vi "GeoData.vi"() -> ()   [LabVIEW 2017] (continued)
H1\n44202\t39133\tAurora\tOH\tPortage County\tH1\n44491\t39133\tWest farmington\tOH\tPortage County\tH1\n44201\t39133\tAtwater\tOH\tPortage County\tH1\n44601\t39133\tAlliance\tOH\tPortage County\tH1\n44412\t39133\tDiamond\tOH\tPortage County\tH1\n44265\t39133\tRandolph\tOH\tPortage County\tH1\n44255\t39133\tMantua\tOH\tPortage County\tH1\n44231\t39133\tGarrettsville\tOH\tPortage County\tH1\n44288\t39133\tWindham\tOH\tPortage County\tH1\n44312\t39133\tAkron\tOH\tPortage County\tH1\n44429\t39133\tLake milton\tOH\tPortage County\tH1\n44632\t39133\tHartville\tOH\tPortage County\tH1\n44234\t39133\tHiram\tOH\tPortage County\tH1\n44224\t39133\tStow\tOH\tPortage County\tH1\n44444\t39133\tNewton falls\tOH\tPortage County\tH1\n44470\t39133\tSouthington\tOH\tPortage County\tH1\n44411\t39133\tDeerfield\tOH\tPortage County\tH1\n45003\t39135\tCollege corner\tOH\tPreble County\tH1\n45304\t39135\tArcanum\tOH\tPreble County\tH1\n45382\t39135\tWest manchester\tOH\tPreble County\tH1\n45311\t39135\tCamden\tOH\tPreble County\tH1\n45338\t39135\tLewisburg\tOH\tPreble County\tH1\n45309\t39135\tBrookville\tOH\tPreble County\tH1\n45327\t39135\tGermantown\tOH\tPreble County\tH1\n45381\t39135\tWest alexandria\tOH\tPreble County\tH1\n45064\t39135\tSomerville\tOH\tPreble County\tH1\n45320\t39135\tEaton\tOH\tPreble County\tH1\n45347\t39135\tNew paris\tOH\tPreble County\tH1\n45378\t39135\tVerona\tOH\tPreble County\tH1\n45070\t39135\tWest elkton\tOH\tPreble County\tH1\n45042\t39135\tMiddletown\tOH\tPreble County\tH1\n45056\t39135\tOxford\tOH\tPreble County\tH1\n45325\t39135\tFarmersville\tOH\tPreble County\tH1\n45321\t39135\tEldorado\tOH\tPreble County\tH1\n45330\t39135\tGratis\tOH\tPreble County\tH1\n45830\t39137\tColumbus grove\tOH\tPutnam County\tH1\n45858\t39137\tMc comb\tOH\tPutnam County\tH1\n45837\t39137\tDupont\tOH\tPutnam County\tH1\n45807\t39137\tLima\tOH\tPutnam County\tH1\n45873\t39137\tOakwood\tOH\tPutnam County\tH1\n45877\t39137\tPandora\tOH\tPutnam County\tH1\n45831\t39137\tContinental\tOH\tPutnam County\tH1\n45853\t39137\tKalida\tOH\tPutnam County\tH1\n43548\t39137\tNew bavaria\tOH\tPutnam County\tH1\n45849\t39137\tGrover hill\tOH\tPutnam County\tH1\n45827\t39137\tCloverdale\tOH\tPutnam County\tH1\n45876\t39137\tOttoville\tOH\tPutnam County\tH1\n45848\t39137\tGlandorf\tOH\tPutnam County\tH1\n43516\t39137\tDeshler\tOH\tPutnam County\tH1\n45833\t39137\tDelphos\tOH\tPutnam County\tH1\n45856\t39137\tLeipsic\tOH\tPutnam County\tH1\n45844\t39137\tFort jennings\tOH\tPutnam County\tH1\n45893\t39137\tVaughnsville\tOH\tPutnam County\tH1\n45817\t39137\tBluffton\tOH\tPutnam County\tH1\n45868\t39137\tMount cory\tOH\tPutnam County\tH1\n45864\t39137\tMiller city\tOH\tPutnam County\tH1\n45875\t39137\tOttawa\tOH\tPutnam County\tH1\n44827\t39139\tCrestline\tOH\tRichland County\tH1\n44902\t39139\tMansfield\tOH\tRichland County\tH1\n44843\t39139\tLucas\tOH\tRichland County\tH1\n44864\t39139\tPerrysville\tOH\tRichland County\tH1\n44901\t39139\tMansfield\tOH\tRichland County\tH1\n44805\t39139\tAshland\tOH\tRichland County\tH1\n44906\t39139\tMansfield\tOH\tRichland County\tH1\n44837\t39139\tGreenwich\tOH\tRichland County\tH1\n44875\t39139\tShelby\tOH\tRichland County\tH1\n44905\t39139\tMansfield\tOH\tRichland County\tH1\n44822\t39139\tButler\tOH\tRichland County\tH1\n44903\t39139\tMansfield\tOH\tRichland County\tH1\n44878\t39139\tShiloh\tOH\tRichland County\tH1\n44907\t39139\tMansfield\tOH\tRichland County\tH1\n44904\t39139\tMansfield\tOH\tRichland County\tH1\n44865\t39139\tPlymouth\tOH\tRichland County\tH1\n44862\t39139\tOntario\tOH\tRichland County\tH1\n44833\t39139\tGalion\tOH\tRichland County\tH1\n44813\t39139\tBellville\tOH\tRichland County\tH1\n43019\t39139\tFredericktown\tOH\tRichland County\tH1\n45601\t39141\tChillicothe\tOH\tRoss County\tH1\n45690\t39141\tWaverly\tOH\tRoss County\tH1\n45628\t39141\tFrankfort\tOH\tRoss County\tH1\n43115\t39141\tClarksburg\tOH\tRoss County\tH1\n45673\t39141\tRichmond dale\tOH\tRoss County\tH1\n43101\t39141\tAdelphi\tOH\tRoss County\tH1\n45123\t39141\tGreenfield\tOH\tRoss County\tH1\n43164\t39141\tWilliamsport\tOH\tRoss County\tH1\n45647\t39141\tLondonderry\tOH\tRoss County\tH1\n43160\t39141\tWashington court house\tOH\tRoss County\tH1\n45644\t39141\tKingston\tOH\tRoss County\tH1\n45672\t39141\tRay\tOH\tRoss County\tH1\n45633\t39141\tHallsville\tOH\tRoss County\tH1\n43135\t39141\tLaurelville\tOH\tRoss County\tH1\n45612\t39141\tBainbridge\tOH\tRoss County\tH1\n45681\t39141\tSouth salem\tOH\tRoss County\tH1\n45617\t39141\tBourneville\tOH\tRoss County\tH1\n44824\t39143\tCastalia\tOH\tSandusky County\tH1\n43416\t39143\tElmore\tOH\tSandusky County\tH1\n43410\t39143\tClyde\tOH\tSandusky County\tH1\n43431\t39143\tGibsonburg\tOH\tSandusky County\tH1\n43449\t39143\tOak harbor\tOH\tSandusky County\tH1\n43406\t39143\tBradner\tOH\tSandusky County\tH1\n43457\t39143\tRisingsun\tOH\tSandusky County\tH1\n43435\t39143\tHelena\tOH\tSandusky County\tH1\n43464\t39143\tVickery\tOH\tSandusky County\tH1\n44811\t39143\tBellevue\tOH\tSandusky County\tH1\n43469\t39143\tWoodville\tOH\tSandusky County\tH1\n44836\t39143\tGreen springs\tOH\tSandusky County\tH1\n43443\t39143\tLuckey\tOH\tSandusky County\tH1\n43407\t39143\tBurgoon\tOH\tSandusky County\tH1\n43450\t39143\tPemberville\tOH\tSandusky County\tH1\n43430\t39143\tGenoa\tOH\tSandusky County\tH1\n44841\t39143\tKansas\tOH\tSandusky County\tH1\n43420\t39143\tFremont\tOH\tSandusky County\tH1\n43442\t39143\tLindsey\tOH\tSandusky County\tH1\n45660\t39145\tPeebles\tOH\tScioto County\tH1\n45694\t39145\tWheelersburg\tOH\tScioto County\tH1\n45638\t39145\tIronton\tOH\tScioto County\tH1\n45636\t39145\tHaverhill\tOH\tScioto County\tH1\n45699\t39145\tLucasville\tOH\tScioto County\tH1\n45648\t39145\tLucasville\tOH\tScioto County\tH1\n45652\t39145\tMc dermott\tOH\tScioto County\tH1\n45616\t39145\tBlue creek\tOH\tScioto County\tH1\n45629\t39145\tFranklin furnace\tOH\tScioto County\tH1\n45659\t39145\tPedro\tOH\tScioto County\tH1\n45662\t39145\tPortsmouth\tOH\tScioto County\tH1\n45663\t39145\tWest portsmouth\tOH\tScioto County\tH1\n45684\t39145\tStout\tOH\tScioto County\tH1\n45653\t39145\tMinford\tOH\tScioto County\tH1\n45656\t39145\tOak hill\tOH\tScioto County\tH1\n45640\t39145\tJackson\tOH\tScioto County\tH1\n45661\t39145\tPiketon\tOH\tScioto County\tH1\n45682\t39145\tSouth webster\tOH\tScioto County\tH1\n45671\t39145\tRarden\tOH\tScioto County\tH1\n45677\t39145\tScioto furnace\tOH\tScioto County\tH1\n45613\t39145\tBeaver\tOH\tScioto County\tH1\n45657\t39145\tOtway\tOH\tScioto County\tH1\n45630\t39145\tFriendship\tOH\tScioto County\tH1\n44853\t39147\tNew riegel\tOH\tSeneca County\tH1\n43410\t39147\tClyde\tOH\tSeneca County\tH1\n43457\t39147\tRisingsun\tOH\tSeneca County\tH1\n44818\t39147\tBloomville\tOH\tSeneca County\tH1\n44807\t39147\tAttica\tOH\tSeneca County\tH1\n44811\t39147\tBellevue\tOH\tSeneca County\tH1\n44802\t39147\tAlvada\tOH\tSeneca County\tH1\n44830\t39147\tFostoria\tOH\tSeneca County\tH1\n44867\t39147\tRepublic\tOH\tSeneca County\tH1\n44836\t39147\tGreen springs\tOH\tSeneca County\tH1\n44861\t39147\tOld fort\tOH\tSeneca County\tH1\n44809\t39147\tBascom\tOH\tSeneca County\tH1\n44883\t39147\tTiffin\tOH\tSeneca County\tH1\n44854\t39147\tNew washington\tOH\tSeneca County\tH1\n44882\t39147\tSycamore\tOH\tSeneca County\tH1\n44841\t39147\tKansas\tOH\tSeneca County\tH1\n44844\t39147\tMc cutchenville\tOH\tSeneca County\tH1\n44828\t39147\tFlat rock\tOH\tSeneca County\tH1\n43316\t39147\tCarey\tOH\tSeneca County\tH1\n44815\t39147\tBettsville\tOH\tSeneca County\tH1\n44845\t39147\tMelmore\tOH\tSeneca County\tH1\n45865\t39149\tMinster\tOH\tShelby County\tH1\n45363\t39149\tRussia\tOH\tShelby County\tH1\n45333\t39149\tHouston\tOH\tShelby County\tH1\n45340\t39149\tMaplewood\tOH\tShelby County\tH1\n45326\t39149\tFletcher\tOH\tShelby County\tH1\n45306\t39149\tBotkins\tOH\tShelby County\tH1\n45317\t39149\tConover\tOH\tShelby County\tH1\n45336\t39149\tKettlersville\tOH\tShelby County\tH1\n45895\t39149\tWapakoneta\tOH\tShelby County\tH1\n45871\t39149\tNew knoxville\tOH\tShelby County\tH1\n45869\t39149\tNew bremen\tOH\tShelby County\tH1\n45388\t39149\tYorkshire\tOH\tShelby County\tH1\n43343\t39149\tQuincy\tOH\tShelby County\tH1\n45353\t39149\tPemberton\tOH\tShelby County\tH1\n45334\t39149\tJackson center\tOH\tShelby County\tH1\n45380\t39149\tVersailles\tOH\tShelby County\tH1\n45365\t39149\tSidney\tOH\tShelby County\tH1\n45360\t39149\tPort jefferson\tOH\tShelby County\tH1\n45367\t39149\tSidney\tOH\tShelby County\tH1\n45845\t39149\tFort loramie\tOH\tShelby County\tH1\n45302\t39149\tAnna\tOH\tShelby County\tH1\n45356\t39149\tPiqua\tOH\tShelby County\tH1\n44216\t39151\tClinton\tOH\tStark County\tH1\n44706\t39151\tCanton\tOH\tStark County\tH1\n44657\t39151\tMinerva\tOH\tStark County\tH1\n44708\t39151\tCanton\tOH\tStark County\tH1\n44648\t39151\tMassillon\tOH\tStark County\tH1\n44260\t39151\tMogadore\tOH\tStark County\tH1\n44669\t39151\tParis\tOH\tStark County\tH1\n44643\t39151\tMagnolia\tOH\tStark County\tH1\n44718\t39151\tCanton\tOH\tStark County\tH1\n44704\t39151\tCanton\tOH\tStark County\tH1\n44608\t39151\tBeach city\tOH\tStark County\tH1\n44705\t39151\tCanton\tOH\tStark County\tH1\n44702\t39151\tCanton\tOH\tStark County\tH1\n44666\t39151\tNorth lawrence\tOH\tStark County\tH1\n44640\t39151\tLimaville\tOH\tStark County\tH1\n44799\t39151\tCanton\tOH\tStark County\tH1\n44720\t39151\tNorth canton\tOH\tStark County\tH1\n44634\t39151\tHomeworth\tOH\tStark County\tH1\n44614\t39151\tCanal fulton\tOH\tStark County\tH1\n44688\t39151\tWaynesburg\tOH\tStark County\tH1\n44689\t39151\tWilmot\tOH\tStark County\tH1\n44735\t39151\tCanton\tOH\tStark County\tH1\n44711\t39151\tCanton\tOH\tStark County\tH1\n44750\t39151\tCanton\tOH\tStark County\tH1\n44613\t39151\tBrewster\tOH\tStark County\tH1\n44709\t39151\tCanton\tOH\tStark County\tH1\n44710\t39151\tCanton\tOH\tStark County\tH1\n44641\t39151\tLouisville\tOH\tStark County\tH1\n44624\t39151\tDundee\tOH\tStark County\tH1\n44647\t39151\tMassillon\tOH\tStark County\tH1\n44685\t39151\tUniontown\tOH\tStark County\tH1\n44721\t39151\tCanton\tOH\tStark County\tH1\n44650\t39151\tMaximo\tOH\tStark County\tH1\n44201\t39151\tAtwater\tOH\tStark County\tH1\n44601\t39151\tAlliance\tOH\tStark County\tH1\n44645\t39151\tMarshallville\tOH\tStark County\tH1\n44646\t39151\tMassillon\tOH\tStark County\tH1\n44703\t39151\tCanton\tOH\tStark County\tH1\n44730\t39151\tEast canton\tOH\tStark County\tH1\n44630\t39151\tGreentown\tOH\tStark County\tH1\n44714\t39151\tCanton\tOH\tStark County\tH1\n44632\t39151\tHartville\tOH\tStark County\tH1\n44612\t39151\tBolivar\tOH\tStark County\tH1\n44626\t39151\tEast sparta\tOH\tStark County\tH1\n44670\t39151\tRobertsville\tOH\tStark County\tH1\n44662\t39151\tNavarre\tOH\tStark County\tH1\n44707\t39151\tCanton\tOH\tStark County\tH1\n44618\t39151\tDalton\tOH\tStark County\tH1\n44680\t39151\tStrasburg\tOH\tStark County\tH1\n44652\t39151\tMiddlebranch\tOH\tStark County\tH1\n44767\t39151\tCanton\tOH\tStark County\tH1\n44304\t39153\tAkron\tOH\tSummit County\tH1\n44216\t39153\tClinton\tOH\tSummit County\tH1\n44314\t39153\tAkron\tOH\tSummit County\tH1\n44087\t39153\tTwinsburg\tOH\tSummit County\tH1\n44056\t39153\tMacedonia\tOH\tSummit County\tH1\n44256\t39153\tMedina\tOH\tSummit County\tH1\n44278\t39153\tTallmadge\tOH\tSummit County\tH1\n44260\t39153\tMogadore\tOH\tSummit County\tH1\n44308\t39153\tAkron\tOH\tSummit County\tH1\n44232\t39153\tGreen\tOH\tSummit County\tH1\n44396\t39153\tAkron\tOH\tSummit County\tH1\n44223\t39153\tCuyahoga falls\tOH\tSummit County\tH1\n44236\t39153\tHudson\tOH\tSummit County\tH1\n44301\t39153\tAkron\tOH\tSummit County\tH1\n44302\t39153\tAkron\tOH\tSummit County\tH1\n44328\t39153\tAkron\tOH\tSummit County\tH1\n44240\t39153\tKent\tOH\tSummit County\tH1\n44202\t39153\tAurora\tOH\tSummit County\tH1\n44230\t39153\tDoylestown\tOH\tSummit County\tH1\n44264\t39153\tPeninsula\tOH\tSummit County\tH1\n44306\t39153\tAkron\tOH\tSummit County\tH1\n44720\t39153\tNorth canton\tOH\tSummit County\tH1\n44614\t39153\tCanal fulton\tOH\tSummit County\tH1\n44250\t39153\tLakemore\tOH\tSummit County\tH1\n44317\t39153\tAkron\tOH\tSummit County\tH1\n44221\t39153\tCuyahoga falls\tOH\tSummit County\tH1\n44305\t39153\tAkron\tOH\tSummit County\tH1\n44141\t39153\tBrecksville\tOH\tSummit County\tH1\n44286\t39153\tRichfield\tOH\tSummit County\tH1\n44262\t39153\tMunroe falls\tOH\tSummit County\tH1\n44320\t39153\tAkron\tOH\tSummit County\tH1\n44313\t39153\tAkron\tOH\tSummit County\tH1\n44685\t39153\tUniontown\tOH\tSummit County\tH1\n44309\t39153\tAkron\tOH\tSummit County\tH1\n44210\t39153\tBath\tOH\tSummit County\tH1\n44303\t39153\tAkron\tOH\tSummit County\tH1\n44310\t39153\tAkron\tOH\tSummit County\tH1\n44307\t39153\tAkron\tOH\tSummit County\tH1\n44311\t39153\tAkron\tOH\tSummit County\tH1\n44067\t39153\tNorthfield\tOH\tSummit County\tH1\n44645\t39153\tMarshallville\tOH\tSummit County\tH1\n44325\t39153\tAkron\tOH\tSummit County\tH1\n44316\t39153\tAkron\tOH\tSummit County\tH1\n44281\t39153\tWadsworth\tOH\tSummit County\tH1\n44333\t39153\tAkron\tOH\tSummit County\tH1\n44312\t39153\tAkron\tOH\tSummit County\tH1\n44321\t39153\tAkron\tOH\tSummit County\tH1\n44222\t39153\tCuyahoga falls\tOH\tSummit County\tH1\n44326\t39153\tAkron\tOH\tSummit County\tH1\n44203\t39153\tBarberton\tOH\tSummit County\tH1\n44224\t39153\tStow\tOH\tSummit County\tH1\n44319\t39153\tAkron\tOH\tSummit County\tH1\n44237\t39153\tHudson\tOH\tSummit County\tH1\n44334\t39153\tFairlawn\tOH\tSummit County\tH1\n44315\t39153\tAkron\tOH\tSummit County\tH1\n44410\t39155\tCortland\tOH\tTrumbull County\tH1\n44430\t39155\tLeavittsburg\tOH\tTrumbull County\tH1\n44418\t39155\tFowler\tOH\tTrumbull County\tH1\n44439\t39155\tMesopotamia\tOH\tTrumbull County\tH1\n44446\t39155\tNiles\tOH\tTrumbull County\tH1\n44484\t39155\tWarren\tOH\tTrumbull County\tH1\n44438\t39155\tMasury\tOH\tTrumbull County\tH1\n44437\t39155\tMc donald\tOH\tTrumbull County\tH1\n44504\t39155\tYoungstown\tOH\tTrumbull County\tH1\n44483\t39155\tWarren\tOH\tTrumbull County\tH1\n44417\t39155\tFarmdale\tOH\tTrumbull County\tH1\n44481\t39155\tWarren\tOH\tTrumbull County\tH1\n44485\t39155\tWarren\tOH\tTrumbull County\tH1\n44491\t39155\tWest farmington\tOH\tTrumbull County\tH1\n44062\t39155\tMiddlefield\tOH\tTrumbull County\tH1\n44424\t39155\tHartford\tOH\tTrumbull County\tH1\n44420\t39155\tGirard\tOH\tTrumbull County\tH1\n44428\t39155\tKinsman\tOH\tTrumbull County\tH1\n44076\t39155\tOrwell\tOH\tTrumbull County\tH1\n44450\t39155\tNorth bloomfield\tOH\tTrumbull County\tH1\n44231\t39155\tGarrettsville\tOH\tTrumbull County\tH1\n44288\t39155\tWindham\tOH\tTrumbull County\tH1\n44425\t39155\tHubbard\tOH\tTrumbull County\tH1\n44440\t39155\tMineral ridge\tOH\tTrumbull County\tH1\n44473\t39155\tVienna\tOH\tTrumbull County\tH1\n44404\t39155\tBurghill\tOH\tTrumbull County\tH1\n44505\t39155\tYoungstown\tOH\tTrumbull County\tH1\n44402\t39155\tBristolville\tOH\tTrumbull County\tH1\n44093\t39155\tWilliamsfield\tOH\tTrumbull County\tH1\n44453\t39155\tOrangeville\tOH\tTrumbull County\tH1\n44444\t39155\tNewton falls\tOH\tTrumbull County\tH1\n44470\t39155\tSouthington\tOH\tTrumbull County\tH1\n44403\t39155\tBrookfield\tOH\tTrumbull County\tH1\n44622\t39157\tDover\tOH\tTuscarawas County\tH1\n43837\t39157\tPort washington\tOH\tTuscarawas County\tH1\n44699\t39157\tTippecanoe\tOH\tTuscarawas County\tH1\n44679\t39157\tStillwater\tOH\tTuscarawas County\tH1\n44656\t39157\tMineral city\tOH\tTuscarawas County\tH1\n44643\t39157\tMagnolia\tOH\tTuscarawas County\tH1\n43824\t39157\tFresno\tOH\tTuscarawas County\tH1\n44608\t39157\tBeach city\tOH\tTuscarawas County\tH1\n43749\t39157\tKimbolton\tOH\tTuscarawas County\tH1\n44621\t39157\tDennison\tOH\tTuscarawas County\tH1\n44681\t39157\tSugarcreek\tOH\tTuscarawas County\tH1\n44653\t39157\tMidvale\tOH\tTuscarawas County\tH1\n43973\t39157\tFreeport\tOH\tTuscarawas County\tH1\n44683\t39157\tUhrichsville\tOH\tTuscarawas County\tH1\n44624\t39157\tDundee\tOH\tTuscarawas County\tH1\n43804\t39157\tBaltic\tOH\tTuscarawas County\tH1\n44663\t39157\tNew philadelphia\tOH\tTuscarawas County\tH1\n44675\t39157\tSherrodsville\tOH\tTuscarawas County\tH1\n43832\t39157\tNewcomerstown\tOH\tTuscarawas County\tH1\n44697\t39157\tZoar\tOH\tTuscarawas County\tH1\n44682\t39157\tTuscarawas\tOH\tTuscarawas County\tH1\n44671\t39157\tSandyville\tOH\tTuscarawas County\tH1\n44612\t39157\tBolivar\tOH\tTuscarawas County\tH1\n44626\t39157\tEast sparta\tOH\tTuscarawas County\tH1\n43840\t39157\tStone creek\tOH\tTuscarawas County\tH1\n44678\t39157\tSomerdale\tOH\tTuscarawas County\tH1\n44680\t39157\tStrasburg\tOH\tTuscarawas County\tH1\n44629\t39157\tGnadenhutten\tOH\tTuscarawas County\tH1\n43064\t39159\tPlain city\tOH\tUnion County\tH1\n43061\t39159\tOstrander\tOH\tUnion County\tH1\n43319\t39159\tEast liberty\tOH\tUnion County\tH1\n43029\t39159\tIrwin\tOH\tUnion County\tH1\n43344\t39159\tRichwood\tOH\tUnion County\tH1\n43345\t39159\tRidgeway\tOH\tUnion County\tH1\n43015\t39159\tDelaware\tOH\tUnion County\tH1\n43067\t39159\tRaymond\tOH\tUnion County\tH1\n43036\t39159\tMagnetic springs\tOH\tUnion County\tH1\n43340\t39159\tMount victory\tOH\tUnion County\tH1\n43302\t39159\tMarion\tOH\tUnion County\tH1\n43060\t39159\tNorth lewisburg\tOH\tUnion County\tH1\n43045\t39159\tMilford center\tOH\tUnion County\tH1\n43077\t39159\tUnionville center\tOH\tUnion County\tH1\n43358\t39159\tWest mansfield\tOH\tUnion County\tH1\n43342\t39159\tProspect\tOH\tUnion County\tH1\n43007\t39159\tBroadway\tOH\tUnion County\tH1\n43040\t39159\tMarysville\tOH\tUnion County\tH1\n43017\t39159\tDublin\tOH\tUnion County\tH1\n43016\t39159\tDublin\tOH\tUnion County\tH1\n43084\t39159\tWoodstock\tOH\tUnion County\tH1\n45832\t39161\tConvoy\tOH\tVan Wert County\tH1\n45838\t39161\tElgin\tOH\tVan Wert County\tH1\n45863\t39161\tMiddle point\tOH\tVan Wert County\tH1\n45849\t39161\tGrover hill\tOH\tVan Wert County\tH1\n45882\t39161\tRockford\tOH\tVan Wert County\tH1\n45898\t39161\tWillshire\tOH\tVan Wert County\tH1\n45833\t39161\tDelphos\tOH\tVan Wert County\tH1\n45844\t39161\tFort jennings\tOH\tVan Wert County\tH1\n45886\t39161\tScott\tOH\tVan Wert County\tH1\n45899\t39161\tWren\tOH\tVan Wert County\tH1\n45894\t39161\tVenedocia\tOH\tVan Wert County\tH1\n45887\t39161\tSpencerville\tOH\tVan Wert County\tH1\n45891\t39161\tVan wert\tOH\tVan Wert County\tH1\n45874\t39161\tOhio city\tOH\tVan Wert County\tH1\n45654\t39163\tNew plymouth\tOH\tVinton County\tH1\n45695\t39163\tWilkesville\tOH\tVinton County\tH1\n45766\t39163\tNew marshfield\tOH\tVinton County\tH1\n45622\t39163\tCreola\tOH\tVinton County\tH1\n45741\t39163\tLangsville\tOH\tVinton County\tH1\n45698\t39163\tZaleski\tOH\tVinton County\tH1\n43138\t39163\tLogan\tOH\tVinton County\tH1\n45686\t39163\tVinton\tOH\tVinton County\tH1\n45634\t39163\tHamden\tOH\tVinton County\tH1\n45651\t39163\tMc arthur\tOH\tVinton County\tH1\n45710\t39163\tAlbany\tOH\tVinton County\tH1\n43152\t39163\tSouth bloomingville\tOH\tVinton County\tH1\n45647\t39163\tLondonderry\tOH\tVinton County\tH1\n45672\t39163\tRay\tOH\tVinton County\tH1\n45692\t39163\tWellston\tOH\tVinton County\tH1\n45005\t39165\tFranklin\tOH\tWarren County\tH1\n45249\t39165\tCincinnati\tOH\tWarren County\tH1\n45342\t39165\tMiamisburg\tOH\tWarren County\tH1\n45162\t39165\tPleasant plain\tOH\tWarren County\tH1\n45066\t39165\tSpringboro\tOH\tWarren County\tH1\n45034\t39165\tKings mills\tOH\tWarren County\tH1\n45040\t39165\tMason\tOH\tWarren County\tH1\n45327\t39165\tGermantown\tOH\tWarren County\tH1\n45107\t39165\tBlanchester\tOH\tWarren County\tH1\n45065\t39165\tSouth lebanon\tOH\tWarren County\tH1\n45152\t39165\tMorrow\tOH\tWarren County\tH1\n45122\t39165\tGoshen\tOH\tWarren County\tH1\n45068\t39165\tWaynesville\tOH\tWarren County\tH1\n45113\t39165\tClarksville\tOH\tWarren County\tH1\n45042\t39165\tMiddletown\tOH\tWarren County\tH1\n45044\t39165\tMiddletown\tOH\tWarren County\tH1\n45050\t39165\tMonroe\tOH\tWarren County\tH1\n45036\t39165\tLebanon\tOH\tWarren County\tH1\n45458\t39165\tDayton\tOH\tWarren County\tH1\n45054\t39165\tOregonia\tOH\tWarren County\tH1\n45032\t39165\tHarveysburg\tOH\tWarren County\tH1\n45039\t39165\tMaineville\tOH\tWarren County\tH1\n45140\t39165\tLoveland\tOH\tWarren County\tH1\n45241\t39165\tCincinnati\tOH\tWarren County\tH1\n43787\t39167\tStockport\tOH\tWashington County\tH1\n45715\t39167\tBeverly\tOH\tWashington County\tH1\n45727\t39167\tDexter city\tOH\tWashington County\tH1\n45746\t39167\tMacksburg\tOH\tWashington County\tH1\n45744\t39167\tLowell\tOH\tWashington County\tH1\n45723\t39167\tCoolville\tOH\tWashington County\tH1\n45721\t39167\tCoal run\tOH\tWashington County\tH1\n45714\t39167\tBelpre\tOH\tWashington County\tH1\n45767\t39167\tNew matamoras\tOH\tWashington County\tH1\n45711\t39167\tAmesville\tOH\tWashington County\tH1\n45734\t39167\tGraysville\tOH\tWashington County\tH1\n45786\t39167\tWaterford\tOH\tWashington County\tH1\n45713\t39167\tBartlett\tOH\tWashington County\tH1\n45745\t39167\tLower salem\tOH\tWashington County\tH1\n45729\t39167\tFleming\tOH\tWashington County\tH1\n45712\t39167\tBarlow\tOH\tWashington County\tH1\n45768\t39167\tNewport\tOH\tWashington County\tH1\n45784\t39167\tVincent\tOH\tWashington County\tH1\n45742\t39167\tLittle hocking\tOH\tWashington County\tH1\n45724\t39167\tCutler\tOH\tWashington County\tH1\n45750\t39167\tMarietta\tOH\tWashington County\tH1\n45773\t39167\tReno\tOH\tWashington County\tH1\n45788\t39167\tWhipple\tOH\tWashington County\tH1\n45789\t39167\tWingett run\tOH\tWashington County\tH1\n45787\t39167\tWatertown\tOH\tWashington County\tH1\n44216\t39169\tClinton\tOH\tWayne County\tH1\n44287\t39169\tWest salem\tOH\tWayne County\tH1\n44691\t39169\tWooster\tOH\tWayne County\tH1\n44677\t39169\tSmithville\tOH\tWayne County\tH1\n44627\t39169\tFredericksburg\tOH\tWayne County\tH1\n44276\t39169\tSterling\tOH\tWayne County\tH1\n44217\t39169\tCreston\tOH\tWayne County\tH1\n44666\t39169\tNorth lawrence\tOH\tWayne County\tH1\n44230\t39169\tDoylestown\tOH\tWayne County\tH1\n44676\t39169\tShreve\tOH\tWayne County\tH1\n44614\t39169\tCanal fulton\tOH\tWayne County\tH1\n44624\t39169\tDundee\tOH\tWayne County\tH1\n44273\t39169\tSeville\tOH\tWayne County\tH1\n44645\t39169\tMarshallville\tOH\tWayne County\tH1\n44611\t39169\tBig prairie\tOH\tWayne County\tH1\n44606\t39169\tApple creek\tOH\tWayne County\tH1\n44840\t39169\tJeromesville\tOH\tWayne County\tH1\n44659\t39169\tMount eaton\tOH\tWayne County\tH1\n44214\t39169\tBurbank\tOH\tWayne County\tH1\n44281\t39169\tWadsworth\tOH\tWayne County\tH1\n44638\t39169\tLakeville\tOH\tWayne County\tH1\n44203\t39169\tBarberton\tOH\tWayne County\tH1\n44270\t39169\tRittman\tOH\tWayne County\tH1\n44662\t39169\tNavarre\tOH\tWayne County\tH1\n44667\t39169\tOrrville\tOH\tWayne County\tH1\n44618\t39169\tDalton\tOH\tWayne County\tH1\n44636\t39169\tKidron\tOH\tWayne County\tH1\n43506\t39171\tBryan\tOH\tWilliams County\tH1\n43570\t39171\tWest unity\tOH\tWilliams County\tH1\n43521\t39171\tFayette\tOH\tWilliams County\tH1\n43501\t39171\tAlvordton\tOH\tWilliams County\tH1\n43517\t39171\tEdgerton\tOH\tWilliams County\tH1\n43554\t39171\tPioneer\tOH\tWilliams County\tH1\n43531\t39171\tKunkle\tOH\tWilliams County\tH1\n43512\t39171\tDefiance\tOH\tWilliams County\tH1\n43518\t39171\tEdon\tOH\tWilliams County\tH1\n43502\t39171\tArchbold\tOH\tWilliams County\tH1\n43557\t39171\tStryker\tOH\tWilliams County\tH1\n43505\t39171\tBlakeslee\tOH\tWilliams County\tH1\n43543\t39171\tMontpelier\tOH\tWilliams County\tH1\n43460\t39173\tRossford\tOH\tWood County\tH1\n43403\t39173\tBowling green\tOH\tWood County\tH1\n45858\t39173\tMc comb\tOH\tWood County\tH1\n43451\t39173\tPortage\tOH\tWood County\tH1\n43654\t39173\tToledo\tOH\tWood County\tH1\n43402\t39173\tBowling green\tOH\tWood County\tH1\n43431\t39173\tGibsonburg\tOH\tWood County\tH1\n43619\t39173\tNorthwood\tOH\tWood County\tH1\n43406\t39173\tBradner\tOH\tWood County\tH1\n43457\t39173\tRisingsun\tOH\tWood County\tH1\n43541\t39173\tMilton center\tOH\tWood County\tH1\n43569\t39173\tWeston\tOH\tWood County\tH1\n43465\t39173\tWalbridge\tOH\tWood County\tH1\n43525\t39173\tHaskins\tOH\tWood County\tH1\n43447\t39173\tMillbury\tOH\tWood County\tH1\n43413\t39173\tCygnet\tOH\tWood County\tH1\n43516\t39173\tDeshler\tOH\tWood County\tH1\n44830\t39173\tFostoria\tOH\tWood County\tH1\n43469\t39173\tWoodville\tOH\tWood County\tH1\n43522\t39173\tGrand rapids\tOH\tWood County\tH1\n45872\t39173\tNorth baltimore\tOH\tWood County\tH1\n43466\t39173\tWayne\tOH\tWood County\tH1\n43443\t39173\tLuckey\tOH\tWood County\tH1\n43565\t39173\tTontogany\tOH\tWood County\tH1\n43605\t39173\tToledo\tOH\tWood County\tH1\n43450\t39173\tPemberville\tOH\tWood County\tH1\n43551\t39173\tPerrysburg\tOH\tWood County\tH1\n43430\t39173\tGenoa\tOH\tWood County\tH1\n43552\t39173\tPerrysburg\tOH\tWood County\tH1\n45889\t39173\tVan buren\tOH\tWood County\tH1\n43462\t39173\tRudolph\tOH\tWood County\tH1\n44817\t39173\tBloomdale\tOH\tWood County\tH1\n43437\t39173\tJerry city\tOH\tWood County\tH1\n43441\t39173\tLemoyne\tOH\tWood County\tH1\n43467\t39173\tWest millgrove\tOH\tWood County\tH1\n43511\t39173\tCustar\tOH\tWood County\tH1\n43463\t39173\tStony ridge\tOH\tWood County\tH1\n43414\t39173\tDunbridge\tOH\tWood County\tH1\n45843\t39175\tForest\tOH\tWyandot County\tH1\n44849\t39175\tNevada\tOH\tWyandot County\tH1\n45867\t39175\tMount blanchard\tOH\tWyandot County\tH1\n43359\t39175\tWharton\tOH\tWyandot County\tH1\n43332\t39175\tLa rue\tOH\tWyandot County\tH1\n43337\t39175\tMorral\tOH\tWyandot County\tH1\n44802\t39175\tAlvada\tOH\tWyandot County\tH1\n43351\t39175\tUpper sandusky\tOH\tWyandot County\tH1\n44882\t39175\tSycamore\tOH\tWyandot County\tH1\n44844\t39175\tMc cutchenville\tOH\tWyandot County\tH1\n43323\t39175\tHarpster\tOH\tWyandot County\tH1\n43330\t39175\tKirby\tOH\tWyandot County\tH1\n43316\t39175\tCarey\tOH\tWyandot County\tH1\n74964\t40001\tWatts\tOK\tAdair County\tH1\n74347\t40001\tKansas\tOK\tAdair County\tH1\n74965\t40001\tWestville\tOK\tAdair County\tH1\n74960\t40001\tStilwell\tOK\tAdair County\tH1\n74931\t40001\tBunch\tOK\tAdair County\tH1\n73716\t40003\tAline\tOK\tAlfalfa County\tH1\n73749\t40003\tJet\tOK\tAlfalfa County\tH1\n73741\t40003\tHelena\tOK\tAlfalfa County\tH1\n73728\t40003\tCherokee\tOK\tAlfalfa County\tH1\n73722\t40003\tBurlington\tOK\tAlfalfa County\tH1\n73739\t40003\tGoltry\tOK\tAlfalfa County\tH1\n73726\t40003\tCarmen\tOK\tAlfalfa County\tH1\n73719\t40003\tAmorita\tOK\tAlfalfa County\tH1\n73717\t40003\tAlva\tOK\tAlfalfa County\tH1\n74553\t40005\tKiowa\tOK\tAtoka County\tH1\n74748\t40005\tKenefic\tOK\tAtoka County\tH1\n74729\t40005\tCaddo\tOK\tAtoka County\tH1\n74569\t40005\tStringtown\tOK\tAtoka County\tH1\n73461\t40005\tWapanucka\tOK\tAtoka County\tH1\n73432\t40005\tColeman\tOK\tAtoka County\tH1\n74576\t40005\tWardville\tOK\tAtoka County\tH1\n74538\t40005\tCoalgate\tOK\tAtoka County\tH1\n74727\t40005\tBoswell\tOK\tAtoka County\tH1\n74540\t40005\tDaisy\tOK\tAtoka County\tH1\n74525\t40005\tAtoka\tOK\tAtoka County\tH1\n74560\t40005\tPittsburg\tOK\tAtoka County\tH1\n74555\t40005\tLane\tOK\tAtoka County\tH1\n74533\t40005\tCaney\tOK\tAtoka County\tH1\n73950\t40007\tTurpin\tOK\tBeaver County\tH1\n73931\t40007\tBalko\tOK\tBeaver County\tH1\n73938\t40007\tForgan\tOK\tBeaver County\tH1\n73932\t40007\tBeaver\tOK\tBeaver County\tH1\n73844\t40007\tGate\tOK\tBeaver County\tH1\n73644\t40009\tElk city\tOK\tBeckham County\tH1\n73645\t40009\tErick\tOK\tBeckham County\tH1\n73627\t40009\tCarter\tOK\tBeckham County\tH1\n73662\t40009\tSayre\tOK\tBeckham County\tH1\n73664\t40009\tSentinel\tOK\tBeckham County\tH1\n73666\t40009\tSweetwater\tOK\tBeckham County\tH1\n73673\t40009\tWillow\tOK\tBeckham County\tH1\n73668\t40009\tTexola\tOK\tBeckham County\tH1\n73763\t40011\tOkeene\tOK\tBlaine County\tH1\n73047\t40011\tHinton\tOK\tBlaine County\tH1\n73040\t40011\tGeary\tOK\tBlaine County\tH1\n73755\t40011\tLongdale\tOK\tBlaine County\tH1\n73724\t40011\tCanton\tOK\tBlaine County\tH1\n73744\t40011\tHitchcock\tOK\tBlaine County\tH1\n73747\t40011\tIsabella\tOK\tBlaine County\tH1\n73770\t40011\tSouthard\tOK\tBlaine County\tH1\n73043\t40011\tGreenfield\tOK\tBlaine County\tH1\n73048\t40011\tHydro\tOK\tBlaine County\tH1\n73772\t40011\tWatonga\tOK\tBlaine County\tH1\n74702\t40013\tDurant\tOK\tBryan County\tH1\n74726\t40013\tBokchito\tOK\tBryan County\tH1\n74748\t40013\tKenefic\tOK\tBryan County\tH1\n74729\t40013\tCaddo\tOK\tBryan County\tH1\n74733\t40013\tColbert\tOK\tBryan County\tH1\n74731\t40013\tCartwright\tOK\tBryan County\tH1\n74720\t40013\tAchille\tOK\tBryan County\tH1\n74753\t40013\tPlatter\tOK\tBryan County\tH1\n73449\t40013\tMead\tOK\tBryan County\tH1\n74727\t40013\tBoswell\tOK\tBryan County\tH1\n74723\t40013\tBennington\tOK\tBryan County\tH1\n74701\t40013\tDurant\tOK\tBryan County\tH1\n74730\t40013\tCalera\tOK\tBryan County\tH1\n74741\t40013\tHendrix\tOK\tBryan County\tH1\n74721\t40013\tAlbany\tOK\tBryan County\tH1\n73017\t40015\tCement\tOK\tCaddo County\tH1\n73042\t40015\tGracemont\tOK\tCaddo County\tH1\n73047\t40015\tHinton\tOK\tCaddo County\tH1\n73079\t40015\tPocasset\tOK\tCaddo County\tH1\n73029\t40015\tCyril\tOK\tCaddo County\tH1\n73015\t40015\tCarnegie\tOK\tCaddo County\tH1\n73005\t40015\tAnadarko\tOK\tCaddo County\tH1\n73059\t40015\tMinco\tOK\tCaddo County\tH1\n73006\t40015\tApache\tOK\tCaddo County\tH1\n73053\t40015\tLookeba\tOK\tCaddo County\tH1\n73092\t40015\tVerden\tOK\tCaddo County\tH1\n73048\t40015\tHydro\tOK\tCaddo County\tH1\n73033\t40015\tEakly\tOK\tCaddo County\tH1\n73038\t40015\tFort cobb\tOK\tCaddo County\tH1\n73009\t40015\tBinger\tOK\tCaddo County\tH1\n73001\t40015\tAlbert\tOK\tCaddo County\tH1\n73014\t40017\tCalumet\tOK\tCanadian County\tH1\n73099\t40017\tYukon\tOK\tCanadian County\tH1\n73127\t40017\tOklahoma city\tOK\tCanadian County\tH1\n73128\t40017\tOklahoma city\tOK\tCanadian County\tH1\n73047\t40017\tHinton\tOK\tCanadian County\tH1\n73040\t40017\tGeary\tOK\tCanadian County\tH1\n73179\t40017\tOklahoma city\tOK\tCanadian County\tH1\n73090\t40017\tUnion city\tOK\tCanadian County\tH1\n73078\t40017\tPiedmont\tOK\tCanadian County\tH1\n73762\t40017\tOkarche\tOK\tCanadian County\tH1\n73064\t40017\tMustang\tOK\tCanadian County\tH1\n73022\t40017\tConcho\tOK\tCanadian County\tH1\n73059\t40017\tMinco\tOK\tCanadian County\tH1\n73173\t40017\tOklahoma city\tOK\tCanadian County\tH1\n73036\t40017\tEl reno\tOK\tCanadian County\tH1\n73085\t40017\tYukon\tOK\tCanadian County\tH1\n73142\t40017\tOklahoma city\tOK\tCanadian County\tH1\n73443\t40019\tLone grove\tOK\tCarter County\tH1\n73403\t40019\tArdmore\tOK\tCarter County\tH1\n73436\t40019\tGene autry\tOK\tCarter County\tH1\n73446\t40019\tMadill\tOK\tCarter County\tH1\n73456\t40019\tRingling\tOK\tCarter County\tH1\n73444\t40019\tHennepin\tOK\tCarter County\tH1\n73463\t40019\tWilson\tOK\tCarter County\tH1\n73402\t40019\tArdmore\tOK\tCarter County\tH1\n73433\t40019\tElmore city\tOK\tCarter County\tH1\n73481\t40019\tRatliff city\tOK\tCarter County\tH1\n73453\t40019\tOverbrook\tOK\tCarter County\tH1\n73487\t40019\tTatums\tOK\tCarter County\tH1\n73438\t40019\tHealdton\tOK\tCarter County\tH1\n73458\t40019\tSpringer\tOK\tCarter County\tH1\n73488\t40019\tTussy\tOK\tCarter County\tH1\n73435\t40019\tFox\tOK\tCarter County\tH1\n73401\t40019\tArdmore\tOK\tCarter County\tH1\n73437\t40019\tGraham\tOK\tCarter County\tH1\n74359\t40021\tOaks\tOK\tCherokee County\tH1\n74434\t40021\tFort gibson\tOK\tCherokee County\tH1\n74441\t40021\tHulbert\tOK\tCherokee County\tH1\n74347\t40021\tKansas\tOK\tCherokee County\tH1\n74464\t40021\tTahlequah\tOK\tCherokee County\tH1\n74465\t40021\tTahlequah\tOK\tCherokee County\tH1\n74471\t40021\tWelling\tOK\tCherokee County\tH1\n74962\t40021\tVian\tOK\tCherokee County\tH1\n74364\t40021\tRose\tOK\tCherokee County\tH1\n74457\t40021\tProctor\tOK\tCherokee County\tH1\n74352\t40021\tLocust grove\tOK\tCherokee County\tH1\n74451\t40021\tPark hill\tOK\tCherokee County\tH1\n74452\t40021\tPeggs\tOK\tCherokee County\tH1\n74427\t40021\tCookson\tOK\tCherokee County\tH1\n74960\t40021\tStilwell\tOK\tCherokee County\tH1\n74931\t40021\tBunch\tOK\tCherokee County\tH1\n74444\t40021\tMoodys\tOK\tCherokee County\tH1\n74735\t40023\tFort towson\tOK\tChoctaw County\tH1\n74759\t40023\tSoper\tOK\tChoctaw County\tH1\n74756\t40023\tSawyer\tOK\tChoctaw County\tH1\n74738\t40023\tGrant\tOK\tChoctaw County\tH1\n74727\t40023\tBoswell\tOK\tChoctaw County\tH1\n74760\t40023\tSpencerville\tOK\tChoctaw County\tH1\n74761\t40023\tSwink\tOK\tChoctaw County\tH1\n74764\t40023\tValliant\tOK\tChoctaw County\tH1\n74743\t40023\tHugo\tOK\tChoctaw County\tH1\n73947\t40025\tKeyes\tOK\tCimarron County\tH1\n73933\t40025\tBoise city\tOK\tCimarron County\tH1\n73937\t40025\tFelt\tOK\tCimarron County\tH1\n73946\t40025\tKenton\tOK\tCimarron County\tH1\n73129\t40027\tOklahoma city\tOK\tCleveland County\tH1\n73150\t40027\tOklahoma city\tOK\tCleveland County\tH1\n73111\t40027\tOklahoma city\tOK\tCleveland County\tH1\n74857\t40027\tNewalla\tOK\tCleveland County\tH1\n73153\t40027\tOklahoma city\tOK\tCleveland County\tH1\n73026\t40027\tNorman\tOK\tCleveland County\tH1\n73165\t40027\tOklahoma city\tOK\tCleveland County\tH1\n74878\t40027\tWanette\tOK\tCleveland County\tH1\n73169\t40027\tOklahoma city\tOK\tCleveland County\tH1\n73110\t40027\tOklahoma city\tOK\tCleveland County\tH1\n73139\t40027\tOklahoma city\tOK\tCleveland County\tH1\n73070\t40027\tNorman\tOK\tCleveland County\tH1\n73068\t40027\tNoble\tOK\tCleveland County\tH1\n73149\t40027\tOklahoma city\tOK\tCleveland County\tH1\n73173\t40027\tOklahoma city\tOK\tCleveland County\tH1\n73051\t40027\tLexington\tOK\tCleveland County\tH1\n73019\t40027\tNorman\tOK\tCleveland County\tH1\n73170\t40027\tOklahoma city\tOK\tCleveland County\tH1\n73160\t40027\tOklahoma city\tOK\tCleveland County\tH1\n73189\t40027\tOklahoma city\tOK\tCleveland County\tH1\n73115\t40027\tOklahoma city\tOK\tCleveland County\tH1\n74851\t40027\tMcloud\tOK\tCleveland County\tH1\n73071\t40027\tNorman\tOK\tCleveland County\tH1\n73072\t40027\tNorman\tOK\tCleveland County\tH1\n73135\t40027\tOklahoma city\tOK\tCleveland County\tH1\n74852\t40027\tMacomb\tOK\tCleveland County\tH1\n73020\t40027\tChoctaw\tOK\tCleveland County\tH1\n73069\t40027\tNorman\tOK\tCleveland County\tH1\n73159\t40027\tOklahoma city\tOK\tCleveland County\tH1\n74534\t40029\tCentrahoma\tOK\tCoal County\tH1\n74572\t40029\tTupelo\tOK\tCoal County\tH1\n74556\t40029\tLehigh\tOK\tCoal County\tH1\n74535\t40029\tClarita\tOK\tCoal County\tH1\n74538\t40029\tCoalgate\tOK\tCoal County\tH1\n74871\t40029\tStonewall\tOK\tCoal County\tH1\n74825\t40029\tAllen\tOK\tCoal County\tH1\n73017\t40031\tCement\tOK\tComanche County\tH1\n73503\t40031\tFort sill\tOK\tComanche County\tH1\n73505\t40031\tLawton\tOK\tComanche County\tH1\n73538\t40031\tElgin\tOK\tComanche County\tH1\n73502\t40031\tLawton\tOK\tComanche County\tH1\n73552\t40031\tIndiahoma\tOK\tComanche County\tH1\n73501\t40031\tLawton\tOK\tComanche County\tH1\n73507\t40031\tLawton\tOK\tComanche County\tH1\n73506\t40031\tLawton\tOK\tComanche County\tH1\n73527\t40031\tCache\tOK\tComanche County\tH1\n73540\t40031\tFaxon\tOK\tComanche County\tH1\n73528\t40031\tChattanooga\tOK\tComanche County\tH1\n73082\t40031\tRush springs\tOK\tComanche County\tH1\n73557\t40031\tMedicine park\tOK\tComanche County\tH1\n73572\t40031\tWalters\tOK\tComanche County\tH1\n73006\t40031\tApache\tOK\tComanche County\tH1\n73055\t40031\tMarlow\tOK\tComanche County\tH1\n73543\t40031\tGeronimo\tOK\tComanche County\tH1\n73541\t40031\tFletcher\tOK\tComanche County\tH1\n73567\t40031\tSterling\tOK\tComanche County\tH1\n73531\t40033\tDevol\tOK\tCotton County\tH1\n73562\t40033\tRandlett\tOK\tCotton County\tH1\n73568\t40033\tTemple\tOK\tCotton County\tH1\n73572\t40033\tWalters\tOK\tCotton County\tH1\n74349\t40035\tKetchum\tOK\tCraig County\tH1\n74332\t40035\tBig cabin\tOK\tCraig County\tH1\n74369\t40035\tWelch\tOK\tCraig County\tH1\n74333\t40035\tBluejacket\tOK\tCraig County\tH1\n74331\t40035\tAfton\tOK\tCraig County\tH1\n74354\t40035\tMiami\tOK\tCraig County\tH1\n74330\t40035\tAdair\tOK\tCraig County\tH1\n74016\t40035\tChelsea\tOK\tCraig County\tH1\n74301\t40035\tVinita\tOK\tCraig County\tH1\n74010\t40037\tBristow\tOK\tCreek County\tH1\n74066\t40037\tSapulpa\tOK\tCreek County\tH1\n74421\t40037\tBeggs\tOK\tCreek County\tH1\n74033\t40037\tGlenpool\tOK\tCreek County\tH1\n74067\t40037\tSapulpa\tOK\tCreek County\tH1\n74132\t40037\tTulsa\tOK\tCreek County\tH1\n74041\t40037\tKiefer\tOK\tCreek County\tH1\n74039\t40037\tKellyville\tOK\tCreek County\tH1\n74126\t40037\tTulsa\tOK\tCreek County\tH1\n74038\t40037\tJennings\tOK\tCreek County\tH1\n74071\t40037\tSlick\tOK\tCreek County\tH1\n74046\t40037\tMilfay\tOK\tCreek County\tH1\n74030\t40037\tDrumright\tOK\tCreek County\tH1\n74079\t40037\tStroud\tOK\tCreek County\tH1\n74131\t40037\tTulsa\tOK\tCreek County\tH1\n74047\t40037\tMounds\tOK\tCreek County\tH1\n74107\t40037\tTulsa\tOK\tCreek County\tH1\n74028\t40037\tDepew\tOK\tCreek County\tH1\n74052\t40037\tOilton\tOK\tCreek County\tH1\n74063\t40037\tSand springs\tOK\tCreek County\tH1\n74044\t40037\tMannford\tOK\tCreek County\tH1\n74081\t40037\tTerlton\tOK\tCreek County\tH1\n74859\t40037\tOkemah\tOK\tCreek County\tH1\n74068\t40037\tShamrock\tOK\tCreek County\tH1\n73096\t40039\tWeatherford\tOK\tCuster County\tH1\n73639\t40039\tCuster city\tOK\tCuster County\tH1\n73620\t40039\tArapaho\tOK\tCuster County\tH1\n73626\t40039\tCanute\tOK\tCuster County\tH1\n73024\t40039\tCorn\tOK\tCuster County\tH1\n73601\t40039\tClinton\tOK\tCuster County\tH1\n73048\t40039\tHydro\tOK\tCuster County\tH1\n73650\t40039\tHammon\tOK\tCuster County\tH1\n73625\t40039\tButler\tOK\tCuster County\tH1\n73669\t40039\tThomas\tOK\tCuster County\tH1\n73654\t40039\tLeedey\tOK\tCuster County\tH1\n74964\t40041\tWatts\tOK\tDelaware County\tH1\n74359\t40041\tOaks\tOK\tDelaware County\tH1\n74370\t40041\tWyandotte\tOK\tDelaware County\tH1\n74366\t40041\tSpavinaw\tOK\tDelaware County\tH1\n74368\t40041\tTwin oaks\tOK\tDelaware County\tH1\n74347\t40041\tKansas\tOK\tDelaware County\tH1\n74345\t40041\tGrove\tOK\tDelaware County\tH1\n74364\t40041\tRose\tOK\tDelaware County\tH1\n74331\t40041\tAfton\tOK\tDelaware County\tH1\n74338\t40041\tColcord\tOK\tDelaware County\tH1\n74346\t40041\tJay\tOK\tDelaware County\tH1\n74342\t40041\tEucha\tOK\tDelaware County\tH1\n74301\t40041\tVinita\tOK\tDelaware County\tH1\n74344\t40041\tGrove\tOK\tDelaware County\tH1\n74365\t40041\tSalina\tOK\tDelaware County\tH1\n74343\t40041\tFairland\tOK\tDelaware County\tH1\n73859\t40043\tVici\tOK\tDewey County\tH1\n73835\t40043\tCamargo\tOK\tDewey County\tH1\n73646\t40043\tFay\tOK\tDewey County\tH1\n73667\t40043\tTaloga\tOK\tDewey County\tH1\n73658\t40043\tOakwood\tOK\tDewey County\tH1\n73659\t40043\tPutnam\tOK\tDewey County\tH1\n73663\t40043\tSeiling\tOK\tDewey County\tH1\n73654\t40043\tLeedey\tOK\tDewey County\tH1\n73840\t40045\tFargo\tOK\tEllis County\tH1\n73832\t40045\tArnett\tOK\tEllis County\tH1\n73858\t40045\tShattuck\tOK\tEllis County\tH1\n73843\t40045\tGage\tOK\tEllis County\tH1\n73761\t40047\tNash\tOK\tGarfield County\tH1\n73073\t40047\tOrlando\tOK\tGarfield County\tH1\n73735\t40047\tDrummond\tOK\tGarfield County\tH1\n73753\t40047\tKremlin\tOK\tGarfield County\tH1\n73736\t40047\tFairmont\tOK\tGarfield County\tH1\n73757\t40047\tLucien\tOK\tGarfield County\tH1\n73733\t40047\tDouglas\tOK\tGarfield County\tH1\n73701\t40047\tEnid\tOK\tGarfield County\tH1\n73738\t40047\tGarber\tOK\tGarfield County\tH1\n73742\t40047\tHennessey\tOK\tGarfield County\tH1\n73718\t40047\tAmes\tOK\tGarfield County\tH1\n73754\t40047\tLahoma\tOK\tGarfield County\tH1\n73702\t40047\tEnid\tOK\tGarfield County\tH1\n73056\t40047\tMarshall\tOK\tGarfield County\tH1\n73730\t40047\tCovington\tOK\tGarfield County\tH1\n73727\t40047\tCarrier\tOK\tGarfield County\tH1\n74630\t40047\tBillings\tOK\tGarfield County\tH1\n74640\t40047\tHunter\tOK\tGarfield County\tH1\n73703\t40047\tEnid\tOK\tGarfield County\tH1\n73773\t40047\tWaukomis\tOK\tGarfield County\tH1\n73739\t40047\tGoltry\tOK\tGarfield County\tH1\n73705\t40047\tEnid\tOK\tGarfield County\tH1\n73720\t40047\tBison\tOK\tGarfield County\tH1\n73743\t40047\tHillsdale\tOK\tGarfield County\tH1\n73098\t40049\tWynnewood\t
